vi "Thermistor.vi"(1 "input variable":dbl) -> (0 "output variable":dbl)   [LabVIEW 2023]
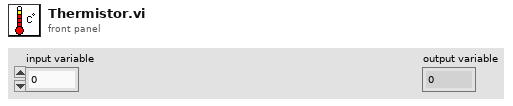
[diagram p1: front panel]
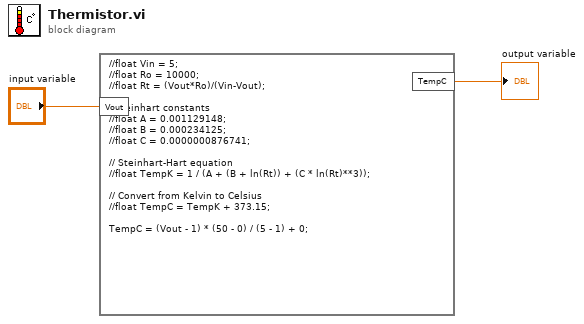
[diagram p0: block diagram]
diagram:
  n1 = formula code="//float Vin = 5;\n//float Ro = 10000;\n//float Rt = (Vout*Ro)/(Vin-Vout);\n\n//Steinhart constants\n//float A = 0.001129148;\n//float B = 0.000234125;\n//float C = 0.0000000876741;\n\n// Steinhart-Hart equation\n//float TempK = 1 / (A + (B + ln(Rt)) + (C * ln(Rt)**3));\n\n// Convert from Kelvin to Celsius\n//float TempC = TempK + 373.15;\n\nTempC = (Vout - 1) * (50 - 0) / (5 - 1) + 0;"("Vout"="input variable") -> ("TempC"=→"output variable":dbl)
